vi "synchronizeDataPlugins.vi"(8 "error in (no error)":errorcluster) -> (0 "error out":errorcluster)   [LabVIEW 2020]
uses:
  <vilib>/Platform/storage/utility/DataPluginSynchronization/_localizeDataPluginMessageEnum.ctl
  <vilib>/Utility/miscctls.llb/LVRowAndColumnUnsignedTypeDef.ctl
  <vilib>/Platform/browser.llb/Open URL in Default Browser (string).vi
  <vilib>/Utility/cursorutil.llb/Set Cursor (Icon Pict).vi
panel:
  in  "Tips":string="Double-click the link in Description to download and install this DataPlugin."
  in  "Close":bool
  in  "Install":bool
  in  "Update All":bool
  in  "DataPlugins":i32[](listbox)
  in  "Search for:":string="Begin with *. to search for file extension only"
  in  "DataPlugin webpage":string="Visit ni.com/dataplugins for detailed information about DataPlugins."
  # "Search DataPlugins by name or file extension:"
  # "Double-click the table headers to sort by Name or Status."
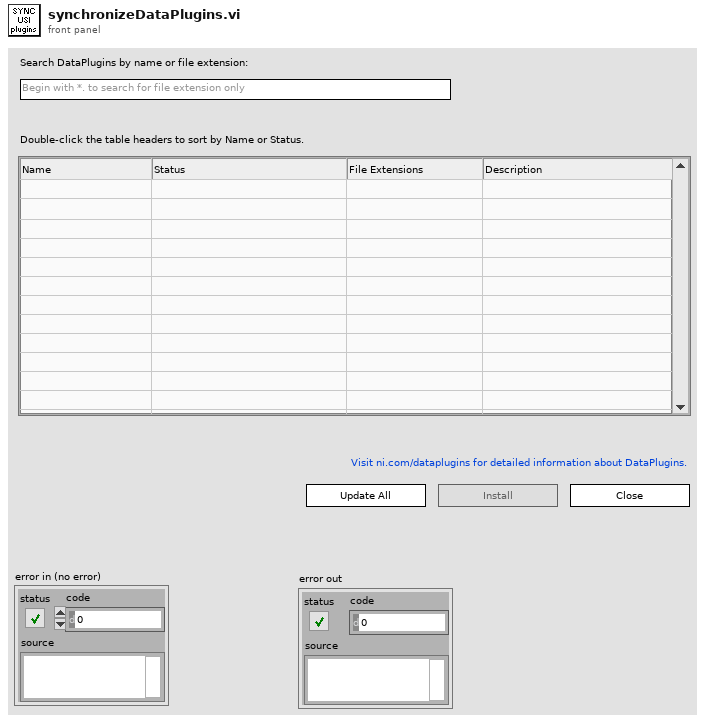
[diagram p1: front panel]
types:
  T1 = enum8{"Enabled", "Disabled", "Disabled and Grayed Out"}
  T2 = typedef "_localizeDataPluginMessageEnum.ctl" = enum16{"Installed", "Not Installed", "Updates Available", "Latest version:", "Double click the \"Description\" cell.", "Install/Update DataPlugins", "Offline: ", "Please ensure that your network connection is working.", "No DataPlugins can be updated.", "Loading DataPlugins from ni.com/dataplugins", "Acquiring and installing ", "Install", "Update", "Succeed", "Failed", " Installation successful.", "Include *. to search for a file extension", "Current version:", " Installation failed.", "Installing update", "Update successful.", "Update failed.", "Updated", "Failed to update DataPlugins."}
  T3 = typedef "_DataPluginInfo.ctl" = cluster{"name":string, "status":u32, "extensions":string[], "description":string, "url":string, "lastExportTime":i64, "type":string, "version":string, "exist":bool, "current version":string, "model":string}
  T4 = typedef "LVRowAndColumnUnsignedTypeDef.ctl" = cluster{"Row":u32, "Column":u32}
  T5 = typedef "LVPoint32TypeDef.ctl" = cluster{"Horizontal":i32, "Vertical":i32}
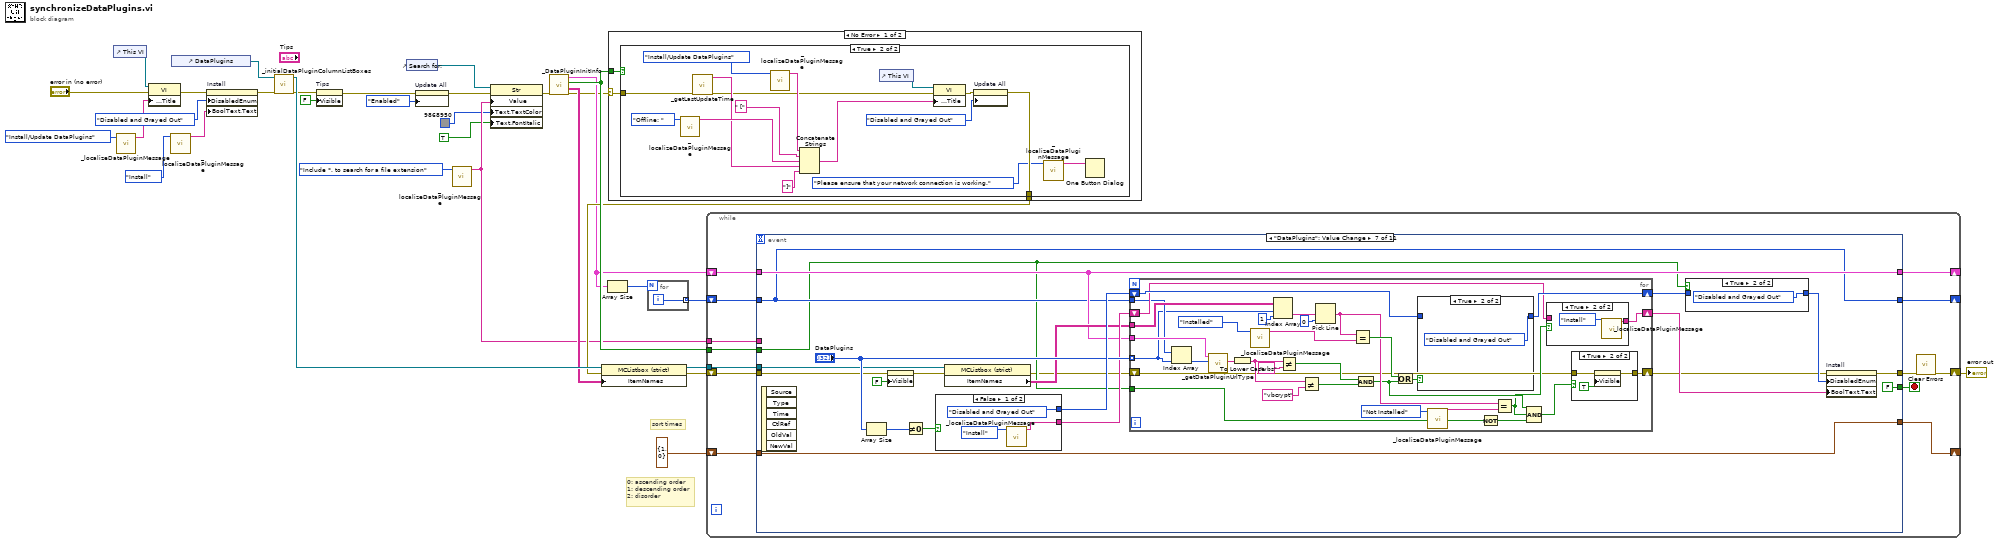
[diagram p0: block diagram]
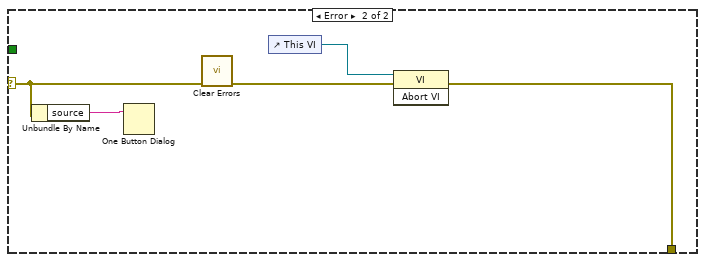
[diagram p3: hidden frame]
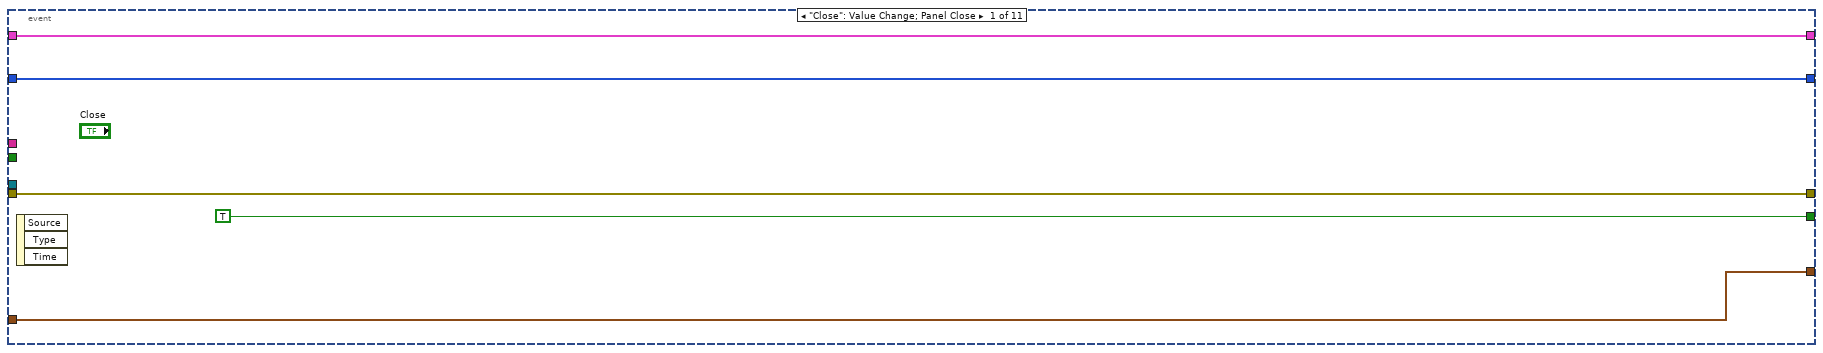
[diagram p4: hidden frame]
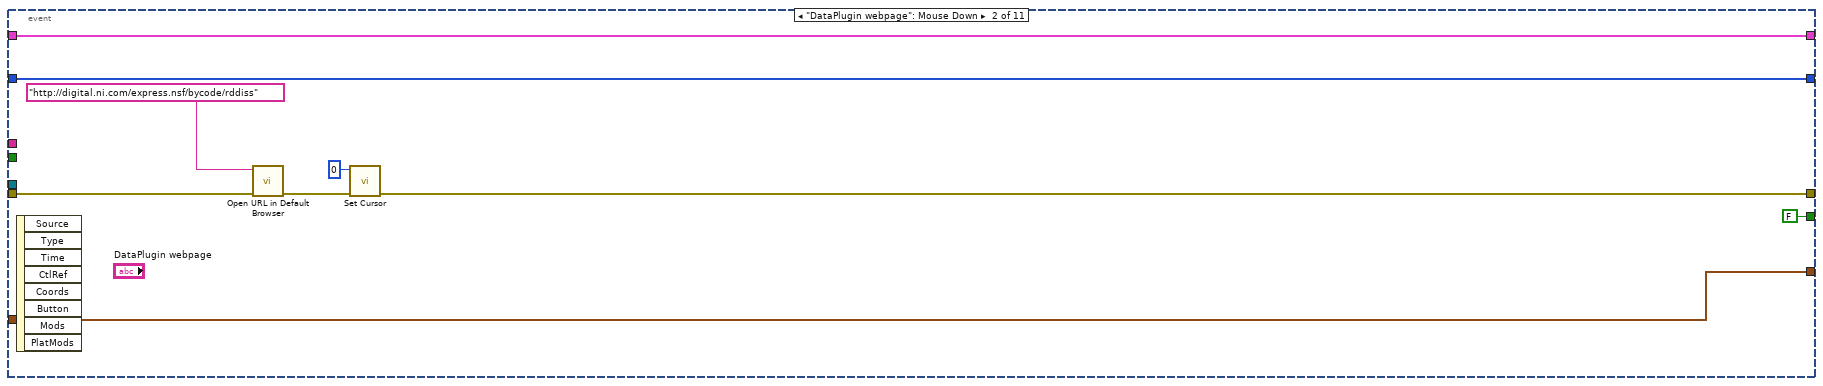
[diagram p5: hidden frame]
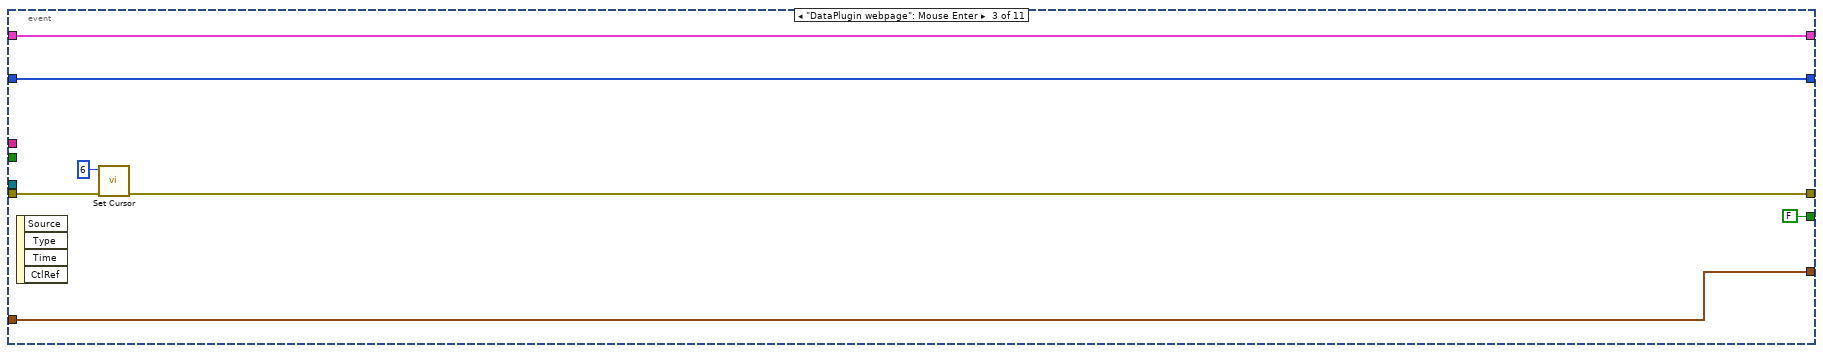
[diagram p6: hidden frame]
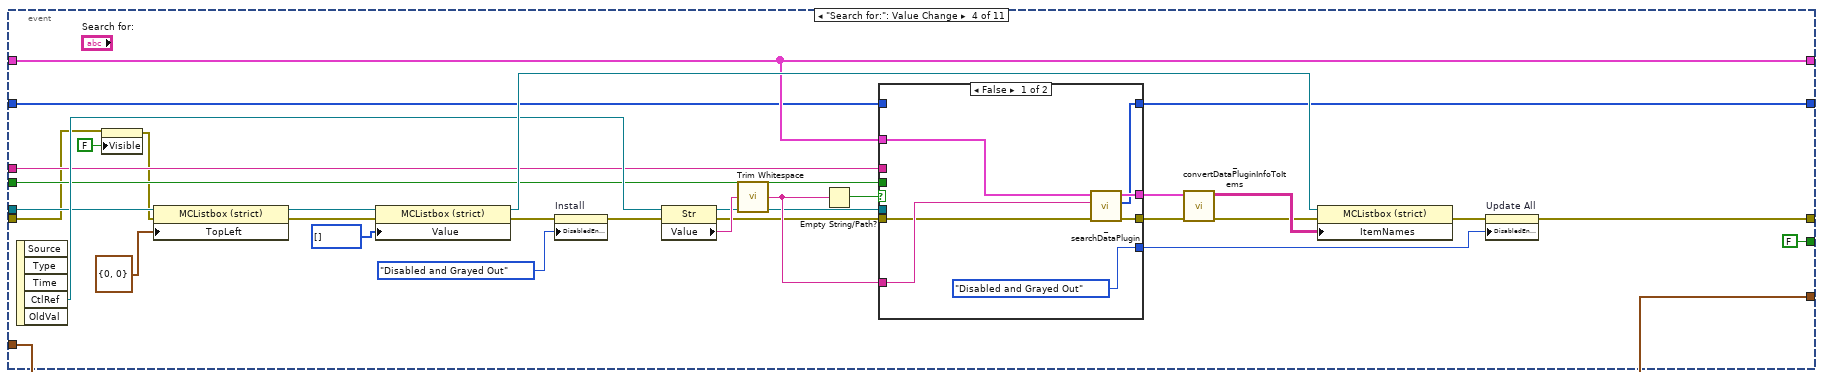
[diagram p7: hidden frame]
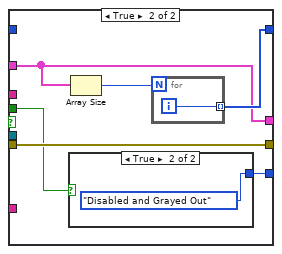
[diagram p8: hidden frame]
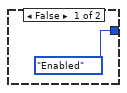
[diagram p9: hidden frame]
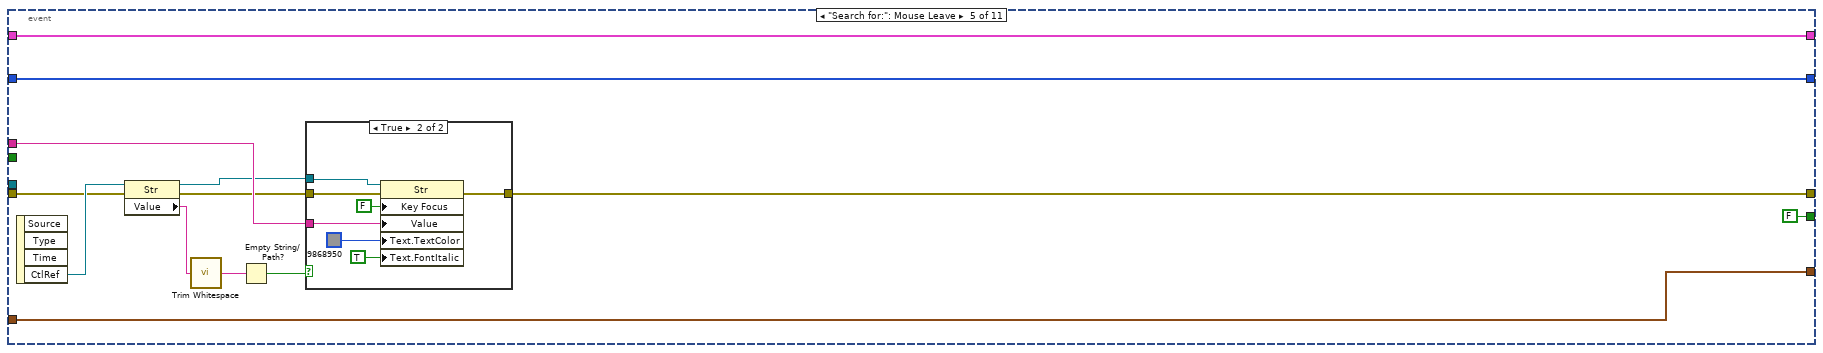
[diagram p10: hidden frame]
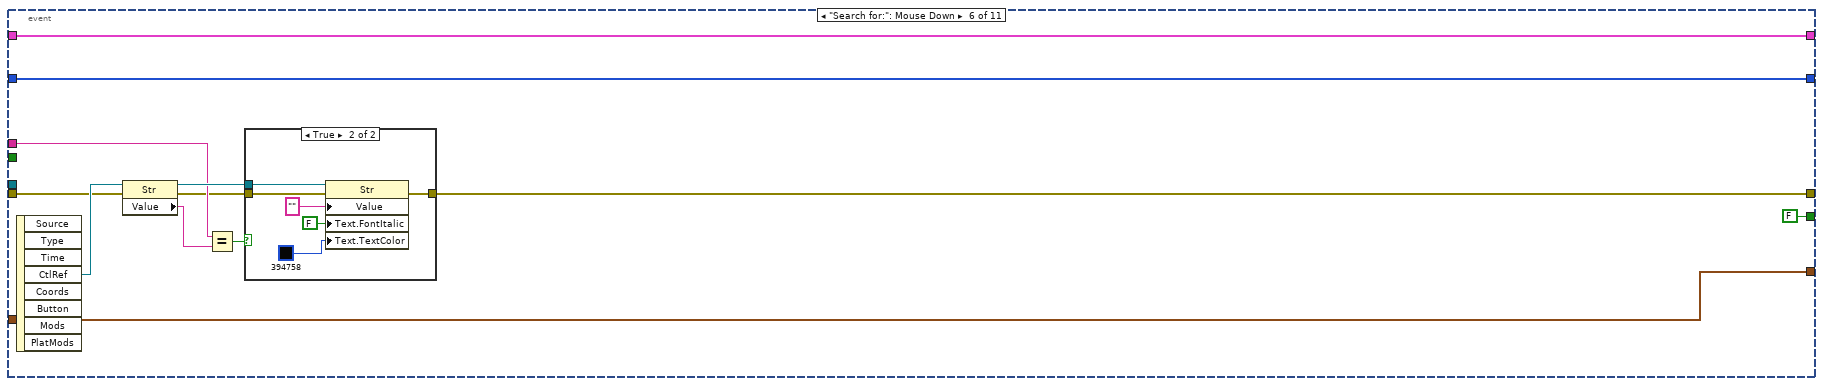
[diagram p12: hidden frame]
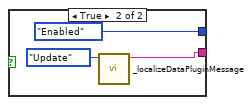
[diagram p15: hidden frame]
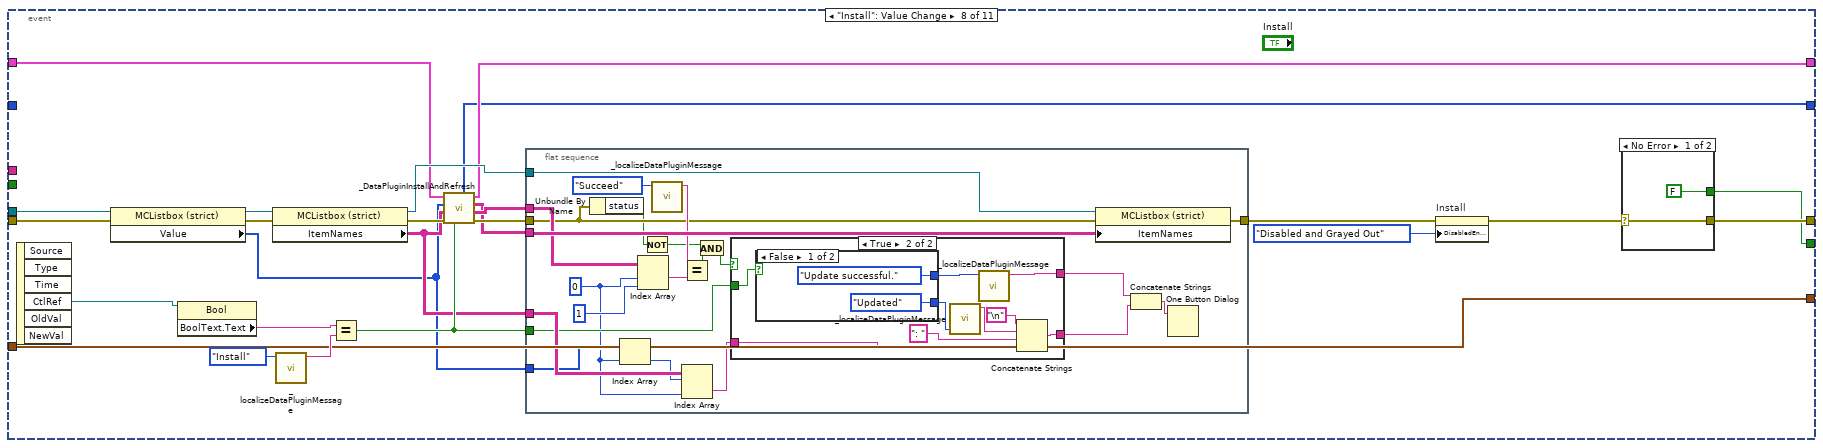
[diagram p19: hidden frame]
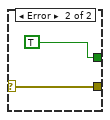
[diagram p20: hidden frame]
diagram:
  # "0: ascending order\n1: descending order\n2: disorder"
  # "sort times"
  n1 = control-ref of="This VI"() -> (w26:refnum<vi>)
  n2 = call <vilib>:"_localizeDataPluginMessage.vi"("message in"=_localizeDataPluginMessageEnum."Install/Update DataPlugins") -> ("message out"=w16:string)  [unwired: 10 in]
  n3 = property class="VI"(reference=w26, error in="error in (no error)", "Front Panel.Title"=w16) -> (error out=w24:errorcluster)  [unwired: 1 out]
  n4 = call <vilib>:"_localizeDataPluginMessage.vi"("message in"=_localizeDataPluginMessageEnum."Install") -> ("message out"=w7:string)  [unwired: 10 in]
  n5 = control-ref of="DataPlugins"() -> (w33:refnum<vi>)
  n6 = property on="Install" class="Bool"(error in=w24, "DisabledEnum"=T1."Disabled and Grayed Out" ("Disabled"), "BoolText.Text"=w7) -> (error out=w23:errorcluster)  [unwired: 1 in, 1 out]
  n7 = call <vilib>:"_initialDataPluginColumnListBoxes.vi"("error in (no error)"=w23, "MulticolumnListbox in"=w33) -> ("error out"=w3:errorcluster, "MulticolumnListbox out"=w31:refnum<vi>)  [unwired: 8 in]
  n8 = property on="Tips" class="Str"(error in=w3, "Visible"=FALSE) -> (error out=w2:errorcluster)  [unwired: 1 in, 1 out]
  n9 = control-ref of="Search for:"() -> (w13:refnum<vi>)
  n10 = property on="Update All" class="Bool"(error in=w2, "DisabledEnum"=T1."Enabled" ("Disabled")) -> (error out=w5:errorcluster)  [unwired: 1 in, 1 out]
  n11 = call <vilib>:"_localizeDataPluginMessage.vi"("message in"=_localizeDataPluginMessageEnum."Include *. to search for a file extension") -> ("message out"=w12:string)  [unwired: 10 in]
  n12 = property class="Str"(reference=w13, error in=w5, "Value"=w12, "Text.TextColor"=u32 9868950, "Text.FontItalic"=TRUE ("Text.Font:Italic")) -> (error out=w9:errorcluster)  [unwired: 1 out]
  n13 = call <vilib>:"_DataPluginInitInfo.vi"("error in (no error)"=w9) -> ("error out"=w4:errorcluster, "Result Items"=w30:string[][], "Offline"=w27:bool, "DataPlugin information out"=w15:T3[])  [unwired: 6 in, 1 out]
  n14 = Array Size(array=w15) -> (size(s)=w14:i32)
  n15 = case shown="No Error" w4 {
    selector: w4 -> [w34 w55]
    tunnel: w27 -> [w36 _]
    tunnel: [w35 w57] -> w22
    frame No Error {
      n16 = case shown="True" w36 {
        tunnel: w34 -> [w37 w39]
        tunnel: [w37 w49] -> w35
        frame False {
        }
        frame True {
          n17 = call <vilib>:"_localizeDataPluginMessage.vi"("message in"=_localizeDataPluginMessageEnum."Offline: ") -> ("message out"=w42:string)  [unwired: 10 in]
          n18 = call <vilib>:"_getLastUpdateTime.vi"("error in (no error)"=w39) -> ("error out"=w38:errorcluster, "LastUpdateTime"=w40:string)  [unwired: 9 in]
          n19 = call <vilib>:"_localizeDataPluginMessage.vi"("message in"=_localizeDataPluginMessageEnum."Install/Update DataPlugins") -> ("message out"=w45:string)  [unwired: 10 in]
          n20 = Concatenate Strings(w45, " [", w42, w40, "]" ("string")) -> (w41:string)
          n21 = control-ref of="This VI"() -> (w53:refnum<vi>)
          n22 = property class="VI"(reference=w53, error in=w38, "Front Panel.Title"=w41) -> (error out=w52:errorcluster)  [unwired: 1 out]
          n23 = property on="Update All" class="Bool"(error in=w52, "DisabledEnum"=T1."Disabled and Grayed Out" ("Disabled")) -> (error out=w49:errorcluster)  [unwired: 1 in, 1 out]
          n24 = call <vilib>:"_localizeDataPluginMessage.vi"("message in"=_localizeDataPluginMessageEnum."Please ensure that your network connection is working.") -> ("message out"=w48:string)  [unwired: 10 in]
          n25 = One Button Dialog(message=w48) -> ()  [unwired: 1 in, 1 out]
        }
      }
    }
    frame Error {
      n26 = Unbundle By Name(w55) -> ("source"=w54:string)
      n27 = One Button Dialog(message=w54) -> ()  [unwired: 1 in, 1 out]
      n28 = call <vilib>:"Clear Errors.vi"("error in (no error)"=w55) -> ("error out"=w56:errorcluster)  [unwired: 5 in, 1 out]
      n29 = control-ref of="This VI"() -> (w58:refnum<vi>)
      n30 = invoke class="VI" method="Abort VI"(reference=w58, error in=w56) -> (error out=w57:errorcluster)  [unwired: 1 in, 2 out]
    }
  }
  n31 = property class="MCListbox (strict)"(reference=w31, error in=w22, "ItemNames"=w30) -> (reference out=w29:refnum<vi>, error out=w32:errorcluster)
  n32 = for {
    N: w14 -> [_]
    tunnel: [w59] -> w18 mode=indexing
    i -> [w59]
  }
  n33 = while {
    shift-right: [w61] -> w28
    shift-left: w32 -> [w71]
    shift-right: [w68] -> _
    shift-left: w15 -> [w70]
    tunnel: w29 -> [w69]
    tunnel: w27 -> [w67]
    tunnel: w12 -> [w66]
    shift-right: [w64] -> _
    shift-left: w18 -> [w65]
    shift-right: [w62] -> _
    shift-left: cluster{i32, i32} {1, 0} -> [w63]
    stop <- w72 stop-if-true
    n34 = event shown="[6] \"DataPlugins\": Value Change" {
      selector: _ -> [_ _ _ _ _ _ _ _ _ _ _]
      dyn-events: _ -> [_ _ _ _ _ _ _ _ _ _ _]
      timeout: _ -> [_ _ _ _ _ _ _ _ _ _ _]
      tunnel: [TRUE FALSE FALSE FALSE FALSE FALSE FALSE w251 w321 FALSE FALSE] -> w72
      tunnel: w71 -> [w75 w85 w93 w96 w144 w165 w184 w267 w328 w365 w465]
      tunnel: w70 -> [w76 w84 w90 w123 w152 w172 w191 w269 w326 w381 w462]
      tunnel: w69 -> [_ _ _ w110 _ _ w195 w268 w330 w366 _]
      tunnel: [w76 w84 w90 w123 w152 w172 w191 w263 w332 w372 w462] -> w68
      tunnel: w67 -> [_ _ _ w104 _ _ w182 _ _ _ _]
      tunnel: w66 -> [_ _ _ w101 w153 w168 _ _ _ _ _]
      tunnel: w65 -> [w74 w83 w88 w106 w147 w171 w190 _ _ w371 w460]
      tunnel: [w74 w83 w88 w105 w147 w171 w190 w250 w320 w370 w460] -> w64
      tunnel: w63 -> [w73 w79 w89 w102 w145 w166 w189 w255 w324 w369 w461]
      tunnel: [w73 w79 w89 w102 w145 w166 w189 w255 w324 w368 w461] -> w62
      tunnel: [w75 w81 w91 w121 w146 w163 w187 w252 w322 w383 w463] -> w60
      event "Close": Value Change; Panel Close {
        n35 = event-data() -> ()  [unwired: 1 in, 3 out]
      }
      event "DataPlugin webpage": Mouse Down {
        n36 = event-data() -> ()  [unwired: 1 in, 8 out]
        n37 = call-poly <vilib>:"Open URL in Default Browser.vi"("error in (no error)"=w85, "URL"="http://digital.ni.com/express.nsf/bycode/rddiss") -> ("error out"=w82:errorcluster)  [unwired: 4 in, 1 out]
        n38 = call-poly <vilib>:"Set Cursor.vi"("error in (no error)"=w82, "icon"=u16 0) -> ("error out"=w81:errorcluster)  [unwired: 8 in, 1 out]
      }
      event "DataPlugin webpage": Mouse Enter {
        n39 = event-data() -> ()  [unwired: 1 in, 4 out]
        n40 = call-poly <vilib>:"Set Cursor.vi"("error in (no error)"=w93, "icon"=u16 6) -> ("error out"=w91:errorcluster)  [unwired: 8 in, 1 out]
      }
      event "Search for:": Value Change {
        n41 = event-data() -> ("CtlRef"=w111:refnum<vi>)  [unwired: 1 in, 4 out]
        n42 = property on="Tips" class="Str"(error in=w96, "Visible"=FALSE) -> (error out=w95:errorcluster)  [unwired: 1 in, 1 out]
        n43 = property class="MCListbox (strict)"(reference=w110, error in=w95, "TopLeft"=T4 {"Row"=0, "Column"=0} ("Top Left Visible Cell")) -> (reference out=w108:refnum<vi>, error out=w109:errorcluster)
        n44 = property class="MCListbox (strict)"(reference=w108, error in=w109, "Value"=i32[] []) -> (reference out=w124:refnum<vi>, error out=w118:errorcluster)
        n45 = property on="Install" class="Bool"(error in=w118, "DisabledEnum"=T1."Disabled and Grayed Out" ("Disabled")) -> (error out=w117:errorcluster)  [unwired: 1 in, 1 out]
        n46 = property on="Property Node" class="Str"(reference=w111, error in=w117) -> (reference out=w99:refnum<vi>, error out=w98:errorcluster, "Value"=w103:string)
        n47 = call <vilib>:"Trim Whitespace.vi"("string"=w103) -> ("trimmed string"=w100:string)  [unwired: 1 in]
        n48 = Empty String/Path?(string/path=w100) -> (empty?=w119:bool)
        n49 = case shown="False" w119 {
          tunnel: w100 -> [w128 _]
          tunnel: w123 -> [w132 w134]
          tunnel: [T1."Disabled and Grayed Out" ("Disabled") w138] -> w120
          tunnel: w98 -> [w127 w137]
          tunnel: [w130 w137] -> w113
          tunnel: [w129 w134] -> w115
          tunnel: w101 -> [_ _]
          tunnel: w99 -> [_ _]
          tunnel: w106 -> [_ _]
          tunnel: [w126 w136] -> w105
          tunnel: w104 -> [_ w135]
          frame False {
            n50 = call <vilib>:"_searchDataPlugin.vi"("error in (no error)"=w127, "Value"=w128, "DataPlugin information"=w132) -> ("error out"=w130:errorcluster, "Indices"=w126:i32[], "DataPlugin information out"=w129:T3[])  [unwired: 6 in]
          }
          frame True {
            n51 = case shown="True" w135 {
              tunnel: [T1."Enabled" ("Disabled") T1."Disabled and Grayed Out" ("Disabled")] -> w138
              frame False {
              }
              frame True {
              }
            }
            n52 = Array Size(array=w134) -> (size(s)=w133:i32)
            n53 = for {
              N: w133 -> [_]
              tunnel: [w141] -> w136 mode=indexing
              i -> [w141]
            }
          }
        }
        n54 = call <vilib>:"_convertDataPluginInfoToItems.vi"("error in (no error)"=w113, "DataPlugin information"=w115) -> ("error out"=w112:errorcluster, "Items"=w114:string[][])  [unwired: 8 in]
        n55 = property class="MCListbox (strict)"(reference=w124, error in=w112, "ItemNames"=w114) -> (error out=w122:errorcluster)  [unwired: 1 out]
        n56 = property on="Update All" class="Bool"(error in=w122, "DisabledEnum"=w120) -> (error out=w121:errorcluster)  [unwired: 1 in, 1 out]
      }
      event "Search for:": Mouse Leave {
        n57 = event-data() -> ("CtlRef"=w151:refnum<vi>)  [unwired: 1 in, 3 out]
        n58 = property class="Str"(reference=w151, error in=w144) -> (error out=w143:errorcluster, "Value"=w150:string)  [unwired: 1 out]
        n59 = call <vilib>:"Trim Whitespace.vi"("string"=w150) -> ("trimmed string"=w149:string)  [unwired: 1 in]
        n60 = Empty String/Path?(string/path=w149) -> (empty?=w148:bool)
        n61 = case shown="True" w148 {
          tunnel: w153 -> [_ w157]
          tunnel: w151 -> [_ w161]
          tunnel: w143 -> [w154 w160]
          tunnel: [w154 w159] -> w146
          frame False {
          }
          frame True {
            n62 = property class="Str"(reference=w161, error in=w160, "Key Focus"=FALSE, "Value"=w157, "Text.TextColor"=u32 9868950, "Text.FontItalic"=TRUE ("Text.Font:Italic")) -> (error out=w159:errorcluster)  [unwired: 1 out]
          }
        }
      }
      event "Search for:": Mouse Down {
        n63 = event-data() -> ("CtlRef"=w170:refnum<vi>)  [unwired: 1 in, 7 out]
        n64 = property class="Str"(reference=w170, error in=w165) -> (error out=w164:errorcluster, "Value"=w169:string)  [unwired: 1 out]
        n65 = Equal?(x=w168, y=w169) -> (x = y?=w167:bool)
        n66 = case shown="True" w167 {
          tunnel: w170 -> [_ w176]
          tunnel: w164 -> [w173 w175]
          tunnel: [w173 w174] -> w163
          frame False {
          }
          frame True {
            n67 = property class="Str"(reference=w176, error in=w175, "Value"="", "Text.FontItalic"=FALSE ("Text.Font:Italic"), "Text.TextColor"=u32 394758) -> (error out=w174:errorcluster)  [unwired: 1 out]
          }
        }
      }
      event "DataPlugins": Value Change {
        n68 = event-data() -> ()  [unwired: 1 in, 6 out]
        n69 = Array Size(array="DataPlugins") -> (size(s)=w198:i32)
        n70 = property on="Tips" class="Str"(error in=w184, "Visible"=FALSE) -> (error out=w183:errorcluster)  [unwired: 1 in, 1 out]
        n71 = Not Equal To 0?(x=w198) -> (x != 0?=w197:bool)
        n72 = case shown="False" w197 {
          tunnel: [T1."Disabled and Grayed Out" ("Disabled") T1."Enabled" ("Disabled")] -> w200
          tunnel: [w204 w207] -> w196
          frame False {
            n73 = call <vilib>:"_localizeDataPluginMessage.vi"("message in"=_localizeDataPluginMessageEnum."Install") -> ("message out"=w204:string)  [unwired: 10 in]
          }
          frame True {
            n74 = call <vilib>:"_localizeDataPluginMessage.vi"("message in"=_localizeDataPluginMessageEnum."Update") -> ("message out"=w207:string)  [unwired: 10 in]
          }
        }
        n75 = property class="MCListbox (strict)"(reference=w195, error in=w183) -> (error out=w181:errorcluster, "ItemNames"=w194:string[][])  [unwired: 1 out]
        n76 = for {
          tunnel: w194 -> [w234]
          tunnel: "DataPlugins" -> [w217] mode=indexing
          shift-right: [w238] -> w193
          shift-left: w200 -> [w237]
          shift-right: [w225] -> w188
          shift-left: w196 -> [w224]
          tunnel: w191 -> [w235]
          tunnel: w190 -> [w218]
          tunnel: w182 -> [w213]
          shift-right: [w209] -> w180
          shift-left: w181 -> [w210]
          n77 = Index Array(array=w218, index=w217) -> (element=w216:i32)
          n78 = call <vilib>:"_getDataPluginUrlType.vi"("DataPlugin Index"=w216, "DataPlugin information"=w235) -> ("type"=w233:string)  [unwired: 8 in, 1 out]
          n79 = To Lower Case(string=w233) -> (all lower case string=w230:string)
          n80 = call <vilib>:"_localizeDataPluginMessage.vi"("message in"=_localizeDataPluginMessageEnum."Installed") -> ("message out"=w221:string)  [unwired: 10 in]
          n81 = Index Array(array=w234, index (row)=w217, index (col)=1 ("disabled index (col)")) -> (element=w236:string)
          n82 = Not Equal?(x=w230, y="vbs") -> (x != y?=w231:bool)
          n83 = Not Equal?(x=w230, y="vbcrypt") -> (x != y?=w228:bool)
          n84 = Pick Line(multi-line string=w236, line index=0) -> (output string=w223:string)  [unwired: 1 in]
          n85 = Equal?(x=w223, y=w221) -> (x = y?=w227:bool)
          n86 = And(x=w231, y=w228) -> (x .and. y?=w215:bool)
          n87 = Or(x=w227, y=w215) -> (x .or. y?=w226:bool)
          n88 = case shown="True" w226 {
            tunnel: [w248 T1."Disabled and Grayed Out" ("Disabled")] -> w238
            tunnel: w237 -> [w248 _]
            frame False {
            }
            frame True {
            }
          }
          n89 = call <vilib>:"_localizeDataPluginMessage.vi"("message in"=_localizeDataPluginMessageEnum."Not Installed") -> ("message out"=w220:string)  [unwired: 10 in]
          n90 = Not(x=w213) -> (.not. x?=w211:bool)
          n91 = Equal?(x=w223, y=w220) -> (x = y?=w214:bool)
          n92 = Compound Arithmetic op=AND(w215, w214, w211) -> (w212:bool)
          n93 = case shown="True" w214 {
            tunnel: w224 -> [w245 _]
            tunnel: [w245 w246] -> w225
            frame False {
            }
            frame True {
              n94 = call <vilib>:"_localizeDataPluginMessage.vi"("message in"=_localizeDataPluginMessageEnum."Install") -> ("message out"=w246:string)  [unwired: 10 in]
            }
          }
          n95 = case shown="True" w212 {
            tunnel: w210 -> [w241 w243]
            tunnel: [w241 w242] -> w209
            frame False {
            }
            frame True {
              n96 = property on="Tips" class="Str"(error in=w243, "Visible"=TRUE) -> (error out=w242:errorcluster)  [unwired: 1 in, 1 out]
            }
          }
        }
        n97 = case shown="True" w182 {
          tunnel: w193 -> [w201 _]
          tunnel: [w201 T1."Disabled and Grayed Out" ("Disabled")] -> w192
          frame False {
          }
          frame True {
          }
        }
        n98 = property on="Install" class="Bool"(error in=w180, "DisabledEnum"=w192, "BoolText.Text"=w188) -> (error out=w187:errorcluster)  [unwired: 1 in, 1 out]
      }
      event "Install": Value Change {
        n99 = event-data() -> ("CtlRef"=w261:refnum<vi>)  [unwired: 1 in, 5 out]
        n100 = property class="MCListbox (strict)"(reference=w268, error in=w267) -> (reference out=w271:refnum<vi>, error out=w274:errorcluster, "Value"=w254:i32[])
        n101 = property class="Bool"(reference=w261) -> ("BoolText.Text"=w260:string)  [unwired: 1 in, 2 out]
        n102 = property class="MCListbox (strict)"(reference=w271, error in=w274) -> (reference out=w270:refnum<vi>, error out=w273:errorcluster, "ItemNames"=w256:string[][])
        n103 = call <vilib>:"_localizeDataPluginMessage.vi"("message in"=_localizeDataPluginMessageEnum."Install") -> ("message out"=w258:string)  [unwired: 10 in]
        n104 = Equal?(x=w260, y=w258) -> (x = y?=w257:bool)
        n105 = call <vilib>:"_DataPluginInstallAndRefresh.vi"("Install?"=w257, "error in"=w273, "Item Names"=w256, "Value"=w254, "DataPlugin Info"=w269) -> ("error out"=w272:errorcluster, "Results"=w264:string[][], "Item Names out"=w262:string[][], "DataPlugin information out"=w263:T3[], "Indices"=w250:i32[])  [unwired: 2 in]
        n106 = flat-sequence {
          tunnel: [w300] -> w266
          tunnel: w262 -> [w299]
          tunnel: w272 -> [w283]
          tunnel: w270 -> [w298]
          tunnel: w264 -> [w297]
          tunnel: w257 -> [w291]
          tunnel: w256 -> [w292]
          tunnel: w254 -> [w288]
          frame #0 {
            w286 = 0 ("disabled index (row)")
            n107 = Unbundle By Name(w283) -> ("status"=w282:bool)
            n108 = Index Array(array=w288, index=w286) -> (element=w287:i32)
            n109 = Index Array(array=w297, index (row)=w286, index (col)=1 ("disabled index (col)")) -> (element=w293:string)
            n110 = Not(x=w282) -> (.not. x?=w281:bool)
            n111 = call <vilib>:"_localizeDataPluginMessage.vi"("message in"=_localizeDataPluginMessageEnum."Succeed") -> ("message out"=w294:string)  [unwired: 10 in]
            n112 = Equal?(x=w294, y=w293) -> (x = y?=w285:bool)
            n113 = Index Array(array=w292, index (row)=w287, index (col)=w286) -> (element=w280:string)
            n114 = And(x=w281, y=w285) -> (x .and. y?=w284:bool)
            n115 = case shown="True" w284 {
              tunnel: [w304 w314] -> w290
              tunnel: w291 -> [w302 w313]
              tunnel: w280 -> [_ w310]
              tunnel: ["" w309] -> w279
              frame False {
                n116 = case shown="False" w302 {
                  tunnel: [_localizeDataPluginMessageEnum."Update failed." ("message in") _localizeDataPluginMessageEnum." Installation failed." ("message in")] -> w303
                  frame False {
                  }
                  frame True {
                  }
                }
                n117 = call <vilib>:"_localizeDataPluginMessage.vi"("message in"=w303) -> ("message out"=w304:string)  [unwired: 10 in]
              }
              frame True {
                n118 = case shown="False" w313 {
                  tunnel: [_localizeDataPluginMessageEnum."Update successful." ("message in") _localizeDataPluginMessageEnum." Installation successful." ("message in")] -> w315
                  tunnel: [_localizeDataPluginMessageEnum."Updated" ("message in") _localizeDataPluginMessageEnum."Installed" ("message in")] -> w312
                  frame False {
                  }
                  frame True {
                  }
                }
                n119 = call <vilib>:"_localizeDataPluginMessage.vi"("message in"=w312) -> ("message out"=w307:string)  [unwired: 10 in]
                n120 = call <vilib>:"_localizeDataPluginMessage.vi"("message in"=w315) -> ("message out"=w314:string)  [unwired: 10 in]
                n121 = Concatenate Strings("\n", w307, ": " ("string"), w310) -> (w309:string)
              }
            }
            n122 = property class="MCListbox (strict)"(reference=w298, error in=w283, "ItemNames"=w299) -> (error out=w300:errorcluster)  [unwired: 1 out]
            n123 = Concatenate Strings(w290, w279) -> (w289:string)
            n124 = One Button Dialog(message=w289) -> ()  [unwired: 1 in, 1 out]
          }
        }
        n125 = property on="Install" class="Bool"(error in=w266, "DisabledEnum"=T1."Disabled and Grayed Out" ("Disabled")) -> (error out=w253:errorcluster)  [unwired: 1 in, 1 out]
        n126 = case shown="No Error" w253 {
          selector: w253 -> [w276 w278]
          tunnel: [w276 w278] -> w252
          tunnel: [FALSE TRUE ("stop? (T)")] -> w251
          frame No Error {
          }
          frame Error {
          }
        }
      }
      event "Update All": Value Change {
        # "2- New version available"
        n127 = event-data() -> ()  [unwired: 1 in, 6 out]
        n128 = call <vilib>:"_convertDataPluginInfoToItems.vi"("error in (no error)"=w328, "DataPlugin information"=w326) -> ("error out"=w327:errorcluster, "Items"=w325:string[][])  [unwired: 8 in]
        n129 = for {
          tunnel: [w344] -> w329 mode=indexing if=w339
          tunnel: w326 -> [w343] mode=indexing
          tunnel: w325 -> [w340] mode=indexing
          tunnel: [w340] -> _ mode=indexing if=w339
          i -> [w344]
          n130 = Unbundle By Name(w343) -> ("status"=w342:u32)
          n131 = Equal?(x=w342, y=u32 2) -> (x = y?=w339:bool)
        }
        n132 = call <vilib>:"_DataPluginInstallAndRefresh.vi"("error in"=w327, "Item Names"=w325, "Value"=w329, "DataPlugin Info"=w326) -> ("error out"=w333:errorcluster, "Results"=w334:string[][], "Item Names out"=w331:string[][], "DataPlugin information out"=w332:T3[], "Indices"=w320:i32[])  [unwired: 3 in]
        n133 = flat-sequence {
          tunnel: [w355] -> w323
          tunnel: w334 -> [w351]
          tunnel: w331 -> [w354]
          tunnel: w333 -> [w347]
          tunnel: w330 -> [w353]
          frame #0 {
            n134 = Unbundle By Name(w347) -> ("status"=w345:bool)
            n135 = Array Size(array=w351) -> (size(s)=w350:i32[])
            n136 = Index Array(array=w350) -> (element=w349:i32)  [unwired: 1 in]
            n137 = Equal To 0?(x=w349) -> (x = 0?=w348:bool)
            n138 = Or(x=w348, y=w345) -> (x .or. y?=w346:bool)
            n139 = case shown="True" w346 {
              tunnel: w351 -> [w358 _]
              tunnel: w347 -> [w357 w359]
              tunnel: [w356 w359] -> w352
              tunnel: w345 -> [_ w362]
              frame False {
                n140 = call <vilib>:"_getInstallationResults.vi"("error in (no error)"=w357, "Item Names"=w358) -> ("error out"=w356:errorcluster)  [unwired: 9 in]
              }
              frame True {
                n141 = case shown="False" w362 {
                  tunnel: [_localizeDataPluginMessageEnum."No DataPlugins can be updated." ("message in") _localizeDataPluginMessageEnum."Failed to update DataPlugins." ("message in")] -> w361
                  frame False {
                  }
                  frame True {
                  }
                }
                n142 = call <vilib>:"_localizeDataPluginMessage.vi"("message in"=w361) -> ("message out"=w360:string)  [unwired: 10 in]
                n143 = One Button Dialog(message=w360) -> ()  [unwired: 1 in, 1 out]
              }
            }
            n144 = property class="MCListbox (strict)"(reference=w353, error in=w352, "ItemNames"=w354) -> (error out=w355:errorcluster)  [unwired: 1 out]
          }
        }
        n145 = case shown="No Error" w323 {
          selector: w323 -> [w336 w338]
          tunnel: [w336 w338] -> w322
          tunnel: [FALSE TRUE ("stop? (T)")] -> w321
          frame No Error {
          }
          frame Error {
          }
        }
      }
      event "DataPlugins": Double Click {
        # "Name"
        n146 = event-data() -> ("Coords"=w380:T5, "Row"=w379:i32)  [unwired: 1 in, 5 out]
        n147 = property class="MCListbox (strict)"(reference=w366, error in=w365) -> (reference out=w375:refnum<vi>, error out=w374:errorcluster, "ItemNames"=w377:string[][])
        n148 = call <vilib>:"_isExpectedDataPluginCell.vi"("Column"=0, "error in (no error)"=w374, "Row"=-1, "Coords"=w380, "MulticolumnListbox"=w375) -> ("error out"=w376:errorcluster, "result"=w373:bool)  [unwired: 5 in]
        n149 = case shown="False" w373 {
          tunnel: [w399 w456] -> w383
          tunnel: w381 -> [w398 w452]
          tunnel: w380 -> [w397 _]
          tunnel: w379 -> [w396 _]
          tunnel: w377 -> [w394 w455]
          tunnel: w376 -> [w393 w458]
          tunnel: w375 -> [w389 w457]
          tunnel: [w388 w451] -> w372
          tunnel: w371 -> [w387 w450]
          tunnel: [w386 w449] -> w370
          tunnel: w369 -> [w385 w447]
          tunnel: [w384 w445] -> w368
          frame False {
            # "Status"
            n150 = call <vilib>:"_isExpectedDataPluginCell.vi"("Column"=1, "error in (no error)"=w393, "Row"=-1, "Coords"=w397, "MulticolumnListbox"=w389) -> ("error out"=w391:errorcluster, "result"=w390:bool)  [unwired: 5 in]
            n151 = case shown="False" w390 {
              tunnel: [w412 w439] -> w399
              tunnel: w398 -> [w404 w437]
              tunnel: w397 -> [w411 _]
              tunnel: w396 -> [w402 _]
              tunnel: w394 -> [w407 w443]
              tunnel: w391 -> [w406 w442]
              tunnel: w389 -> [w405 w440]
              tunnel: [w404 w436] -> w388
              tunnel: w387 -> [w403 w435]
              tunnel: [w403 w434] -> w386
              tunnel: w385 -> [w400 w432]
              tunnel: [w400 w430] -> w384
              frame False {
                # "Description"
                n152 = call <vilib>:"_isExpectedDataPluginCell.vi"("Column"=3, "error in (no error)"=w406, "Row"=w402, "Coords"=w411, "MulticolumnListbox"=w405) -> ("error out"=w409:errorcluster, "result"=w408:bool)  [unwired: 5 in]
                n153 = Index Array(array=w403, index=w402) -> (element=w401:i32)
                n154 = Array Size(array=w407) -> (size(s)=w417:i32[])
                n155 = Index Array(array=w417) -> (element=w416:i32)  [unwired: 1 in]
                n156 = Less?(x=w402, y=w416) -> (x < y?=w414:bool)
                n157 = Greater Or Equal To 0?(x=w402) -> (x >= 0?=w413:bool)
                n158 = Compound Arithmetic op=AND(w408, w414, w413) -> (w415:bool)
                n159 = case shown="True" w415 {
                  tunnel: [w418 w424] -> w412
                  tunnel: w409 -> [w418 w423]
                  tunnel: w404 -> [_ w422]
                  tunnel: w401 -> [_ w419]
                  frame False {
                  }
                  frame True {
                    n160 = call <vilib>:"_getDataPluginUrlType.vi"("DataPlugin Index"=w419, "DataPlugin information"=w422) -> ("Url"=w421:string)  [unwired: 8 in, 1 out]
                    n161 = Empty String/Path?(string/path=w421) -> (empty?=w420:bool)
                    n162 = case shown="False" w420 {
                      tunnel: [w427 w428] -> w424
                      tunnel: w423 -> [w426 w428]
                      tunnel: w421 -> [w425 _]
                      frame False {
                        n163 = call-poly <vilib>:"Open URL in Default Browser.vi"("error in (no error)"=w426, "URL"=w425) -> ("error out"=w427:errorcluster)  [unwired: 4 in, 1 out]
                      }
                      frame True {
                      }
                    }
                  }
                }
              }
              frame True {
                n164 = Unbundle(w432) -> (w433:i32)  [unwired: 1 out]
                n165 = call <vilib>:"_sortItemsByColumnIndex.vi"("times"=w433, "Indices"=w435, "DataPlugin information"=w437, "column Index"=1, "Items in"=w443) -> ("times out"=w431:i32, "Indices out"=w434:i32[], "DataPlugin information out"=w436:T3[], "Items out"=w441:string[][])  [unwired: 3 in]
                n166 = Bundle(cluster=w432, 2, w431) -> (w430:cluster{i32, i32})
                n167 = property class="MCListbox (strict)"(reference=w440, error in=w442, "ItemNames"=w441) -> (error out=w439:errorcluster)  [unwired: 1 out]
              }
            }
          }
          frame True {
            n168 = Unbundle(w447) -> (w448:i32)  [unwired: 1 out]
            n169 = call <vilib>:"_sortItemsByColumnIndex.vi"("times"=w448, "Indices"=w450, "DataPlugin information"=w452, "column Index"=0, "Items in"=w455) -> ("times out"=w446:i32, "Indices out"=w449:i32[], "DataPlugin information out"=w451:T3[], "Items out"=w454:string[][])  [unwired: 3 in]
            n170 = property class="MCListbox (strict)"(reference=w457, error in=w458, "ItemNames"=w454) -> (error out=w456:errorcluster)  [unwired: 1 out]
            n171 = Bundle(cluster=w447, w446, 2) -> (w445:cluster{i32, i32})
          }
        }
      }
      event "DataPlugin webpage": Mouse Leave {
        n172 = event-data() -> ()  [unwired: 1 in, 4 out]
        n173 = call-poly <vilib>:"Set Cursor.vi"("error in (no error)"=w465, "icon"=u16 0) -> ("error out"=w463:errorcluster)  [unwired: 8 in, 1 out]
      }
    }
    n174 = call <vilib>:"Clear Errors.vi"("error in (no error)"=w60) -> ("error out"=w61:errorcluster)  [unwired: 5 in, 1 out]
  }
  "error out" <- w28
